vi "Set Object ACL.vi"(6 "Version ID":string, 7 "AccessControlPolicy":T1, 8 "error in (no error)":errorcluster, 9 "Bucket":string, 10 "Path":string) -> (0 "error out":errorcluster, 3 "PutObjectACLResult":T4)   [LabVIEW 2011, in "LV Interface for Amazon S3.lvlib"]
doc: "This operation <B>sets the access control list (ACL) permissions for an object that already exists</B> in a bucket. (To set the ACL of an object when you put it into a bucket, use Request Parameters' ACL field of the Put Object.vi.) You <B>must have WRITE_ACP permission</B> to set the ACL of an object."
uses:
  LV Interface for Amazon S3.lvlib
  Typedefs/AMZ_S3_API_PUTObjectACLResult.ctl
  Typedefs/AMZ_S3_API_AccessControlPolicy.ctl
  Typedefs/AMZ_S3_API_Owner.ctl
  Typedefs/AMZ_S3_API_Bucket ACL Permission.ctl
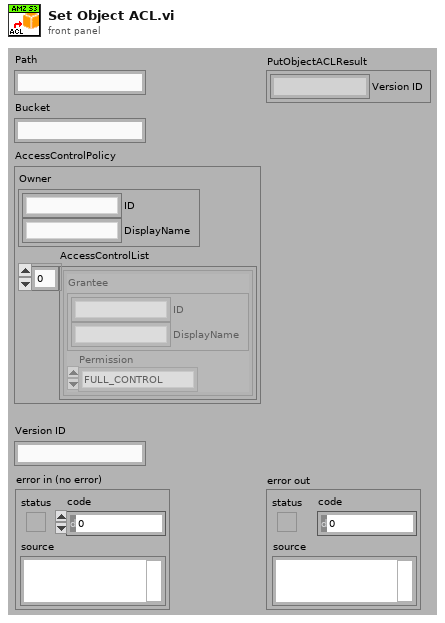
[diagram p1: front panel]
types:
  T1 = typedef "LV Interface for Amazon S3.lvlib/AMZ_S3_API_AccessControlPolicy.ctl" = cluster{"Owner":T2, "AccessControlList":cluster{"Grantee":T2, "Permission":T3}[]}
  T2 = typedef "LV Interface for Amazon S3.lvlib/AMZ_S3_API_Owner.ctl" = cluster{"ID":string, "DisplayName":string}
  T3 = typedef "LV Interface for Amazon S3.lvlib/AMZ_S3_API_Bucket ACL Permission.ctl" = enum16{"FULL_CONTROL", "WRITE", "WRITE_ACP", "READ", "READ_ACP"}
  T4 = typedef "LV Interface for Amazon S3.lvlib/AMZ_S3_API_PUTObjectACLResult.ctl" = cluster{"Version ID":string}
  T5 = typedef "LV Interface for Amazon S3.lvlib/AMZ_S3_Call Results.ctl" = enum16{"Success", "UndefinedError", "AccessDenied", "AccountProblem", "AmbiguousGrantByEmailAddress", "BadDigest", "BucketAlreadyExists", "BucketAlreadyOwnedByYou", "BucketNotEmpty", "CredentialsNotSupported", "CrossLocationLoggingProhibited", "EntityTooSmall", "EntityTooLarge", "ExpiredToken", "IllegalVersioningConfigurationException", "IncompleteBody", "IncorrectNumberOfFilesInPostRequest", "InlineDataTooLarge", "InternalError", "InvalidAccessKeyId", "InvalidAddressingHeader", "InvalidArgument", "InvalidBucketName", "InvalidDigest", "InvalidLocationConstraint", "InvalidPart", "InvalidPartOrder", "InvalidPayer", "InvalidPolicyDocument", "InvalidRange", "InvalidSecurity", "InvalidSOAPRequest", "InvalidStorageClass", "InvalidTargetBucketForLogging", "InvalidToken", "InvalidURI", "KeyTooLong", "MalformedACLError", "MalformedPOSTRequest", "MalformedXML", "MaxMessageLengthExceeded", "MaxPostPreDataLengthExceededError", "MetadataTooLarge", "MethodNotAllowed", "MissingAttachment", "MissingContentLength", "MissingRequestBodyError", "MissingSecurityElement", "MissingSecurityHeader", "NoLoggingStatusForKey", "NoSuchBucket", "NoSuchKey", "NoSuchUpload", "NoSuchVersion", "NotImplemented", "NotSignedUp", "OperationAborted", "PermanentRedirect", "PreconditionFailed", "Redirect", "RequestIsNotMultiPartContent", "RequestTimeout", "RequestTimeTooSkewed", "RequestTorrentOfBucketError", "SignatureDoesNotMatch", "SlowDown", "TemporaryRedirect", "TokenRefreshRequired", "TooManyBuckets", "UnexpectedContent", "UnresolvableGrantByEmailAddress", "UserKeyMustBeSpecified", "LabVIEWError"}
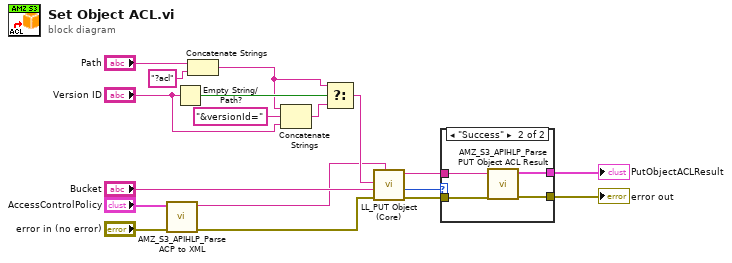
[diagram p0: block diagram]
diagram:
  n1 = call "AMZ_S3_APIHLP_Parse ACP to XML.vi"("error in (no error)"="error in (no error)", "AccessControlPolicy"="AccessControlPolicy") -> ("error out"=w2:errorcluster, "ACP XML String"=w1:string)  [unwired: 8 in]
  n2 = Empty String/Path?(string/path="Version ID") -> (empty?=w12:bool)
  n3 = Concatenate Strings("Path", "?acl" ("string")) -> (w6:string)
  n4 = Concatenate Strings(w6, "&versionId=" ("string"), "Version ID") -> (w10:string)
  n5 = Select(t=w6, s=w12, f=w10) -> (s? t:f=w5:string)
  n6 = call "LL_PUT Object (Core).vi"("Data"=w1, "error in (no error)"=w2, "Bucket"="Bucket", "Path and query string"=w5) -> ("error out"=w16:errorcluster, "Call Result"=w17:T5, "Response header"=w15:string)  [unwired: 4 in, 1 out]
  n7 = case shown="\"Success\"" w17 {
    tunnel: w16 -> [w19 w23]
    tunnel: w15 -> [_ w22]
    tunnel: [_ w21] -> w13
    tunnel: [w19 w20] -> w14
    frame Default {
    }
    frame "Success" {
      n8 = call "AMZ_S3_APIHLP_Parse PUT Object ACL Result.vi"("error in (no error)"=w23, "Response header"=w22) -> ("error out"=w20:errorcluster, "PutObjectACLResult"=w21:T4)  [unwired: 8 in]
    }
  }
  "error out" <- w14
  "PutObjectACLResult" <- w13
